vi "ReadConfigandSetting.vi"(10 "Recipe":string, 11 "Path Out":path) -> (0 "错误输出":errorcluster, 1 "ConfigData":string[][](array[string]), 3 "TableData":string[][](array[string]))   [LabVIEW 2017]
uses:
  <vilib>/Utility/file.llb/Read Delimited Spreadsheet (string).vi
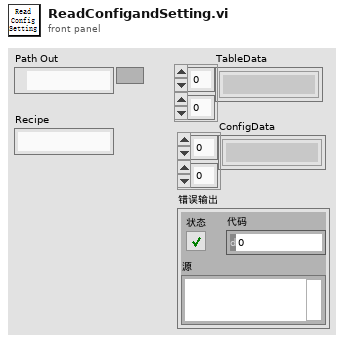
[diagram p1: front panel]
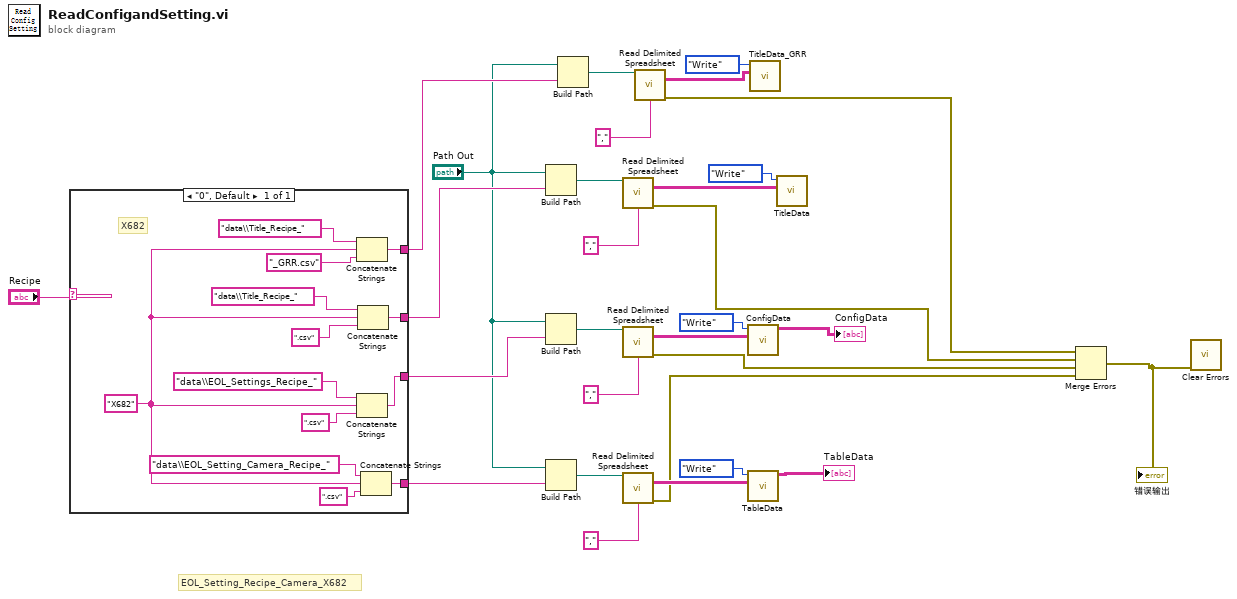
[diagram p0: block diagram]
diagram:
  # "EOL_Setting_Recipe_Camera_X682"
  n1 = case shown="\"0\", Default" "Recipe" {
    tunnel: [w32] -> w10
    tunnel: [w34] -> w11
    tunnel: [w37] -> w12
    tunnel: [w40] -> w13
    frame "0", Default {
      w30 = "X682" ("string")
      # "X682"
      n2 = Concatenate Strings("data\\Title_Recipe_" ("name or relative path"), w30, "_GRR.csv" ("name or relative path")) -> (w40:string)
      n3 = Concatenate Strings("data\\EOL_Settings_Recipe_" ("name or relative path"), w30, ".csv" ("name or relative path")) -> (w34:string)
      n4 = Concatenate Strings("data\\Title_Recipe_" ("name or relative path"), w30, ".csv" ("name or relative path")) -> (w37:string)
      n5 = Concatenate Strings("data\\EOL_Setting_Camera_Recipe_" ("name or relative path"), w30, ".csv" ("name or relative path")) -> (w32:string)
    }
  }
  n6 = Build Path(base path="Path Out", name or relative path=w12) -> (appended path=w26:path)
  n7 = Build Path(base path="Path Out", name or relative path=w11) -> (appended path=w23:path)
  n8 = Build Path(base path="Path Out", name or relative path=w10) -> (appended path=w19:path)
  n9 = Build Path(base path="Path Out", name or relative path=w13) -> (appended path=w17:path)
  n10 = call-poly <vilib>:"Read Delimited Spreadsheet.vi"("file path (dialog if empty)"=w26, "delimiter (\\t)"="," ("delimiter (\\t)")) -> ("all rows"=w28:string[][], "error out"=w4:errorcluster)  [unwired: 8 in, 4 out]
  n11 = call-poly <vilib>:"Read Delimited Spreadsheet.vi"("file path (dialog if empty)"=w23, "delimiter (\\t)"="," ("delimiter (\\t)")) -> ("all rows"=w24:string[][], "error out"=w3:errorcluster)  [unwired: 8 in, 4 out]
  n12 = call-poly <vilib>:"Read Delimited Spreadsheet.vi"("file path (dialog if empty)"=w19, "delimiter (\\t)"="," ("delimiter (\\t)")) -> ("all rows"=w21:string[][], "error out"=w2:errorcluster)  [unwired: 8 in, 4 out]
  n13 = call-poly <vilib>:"Read Delimited Spreadsheet.vi"("file path (dialog if empty)"=w17, "delimiter (\\t)"="," ("delimiter (\\t)")) -> ("all rows"=w15:string[][], "error out"=w5:errorcluster)  [unwired: 8 in, 4 out]
  n14 = call "ConfigData.vi"("Tabledata in"=w24, "Step"=enum16{"Initial", "Write", "Read"}."Write") -> ("Tabledata Out"=→"ConfigData":string[][])  [unwired: 8 in, 1 out]
  n15 = call "TableData.vi"("Tabledata in"=w21, "Step"=enum16{"Initial", "Write", "Read"}."Write") -> ("Tabledata Out"=→"TableData":string[][])  [unwired: 8 in, 1 out]
  n16 = call "TitleData_GRR.vi"("Tabledata in"=w15, "Step"=enum16{"Initial", "Write", "Read"}."Write") -> ()  [unwired: 8 in, 2 out]
  n17 = call "TitleData.vi"("Tabledata in"=w28, "Step"=enum16{"Initial", "Write", "Read"}."Write") -> ()  [unwired: 8 in, 2 out]
  n18 = Merge Errors(w5, w4, w3, w2) -> (w1:errorcluster)
  "错误输出" <- w1
  n19 = call <vilib>:"Clear Errors.vi"("error in (no error)"=w1) -> ()  [unwired: 5 in, 2 out]
